vi "FlatToRichnixnet_grpc_DbGetDatabaseListRequest.vi"(5 "OutputClusterType":T1, 11 "InputCluster":T2) -> (3 "OutputCluster":T1)   [LabVIEW 2025, in "grpc-xnet_client.lvlib"]
uses:
  nixnet_grpc_DbGetDatabaseListRequest_Flat.ctl
  nixnet_grpc_DbGetDatabaseListRequest.ctl
  grpc-xnet_client.lvlib
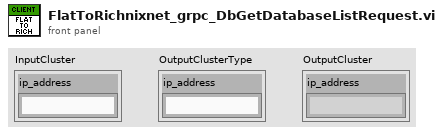
[diagram p1: front panel]
types:
  T1 = typedef "grpc-xnet_client.lvlib/nixnet_grpc_DbGetDatabaseListRequest.ctl" = cluster{"ip_address":string}
  T2 = typedef "grpc-xnet_client.lvlib/nixnet_grpc_DbGetDatabaseListRequest_Flat.ctl" = cluster{"ip_address":string}
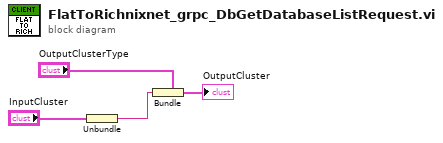
[diagram p0: block diagram]
diagram:
  n1 = Unbundle "Unbundle"("InputCluster") -> ("ip_address"=w1:string)
  n2 = Bundle "Bundle"(cluster="OutputClusterType", "ip_address"=w1) -> (→"OutputCluster":T1)
